vi "F Dwf Analog Out Repeat Info.vi"(7 "pnMax":i32, 8 "error in (no error)":errorcluster, 9 "pnMin":i32, 10 "idxChannel":i32, 11 "hdwf":i32) -> (0 "error out":errorcluster, 1 "pnMin out":i32, 3 "function return":i32, 5 "pnMax out":i32)   [LabVIEW 2021, in "Olasdwf.lvlib"]
doc: "DWFAPI int FDwfAnalogOutRepeatInfo(HDWF hdwf, int idxChannel, int *pnMin, int *pnMax);"
uses:
  Olasdwf.lvlib
  Windows/System32/dwf.dll
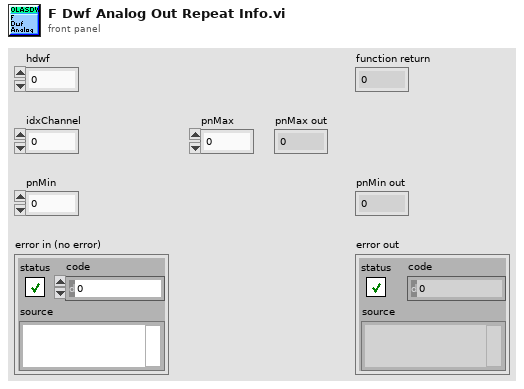
[diagram p1: front panel]
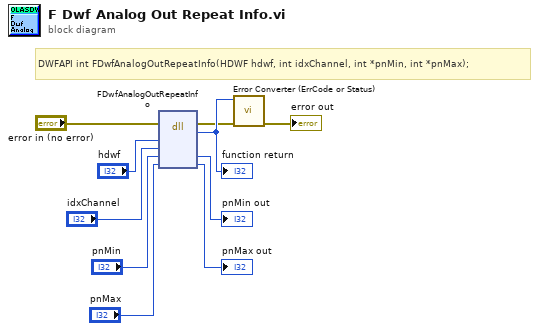
[diagram p0: block diagram]
diagram:
  # "DWFAPI int FDwfAnalogOutRepeatInfo(HDWF hdwf, int idxChannel, int *pnMin, int *pnMax);"
  n1 = dll-call lib="/Windows/System32/dwf.*" fn="FDwfAnalogOutRepeatInfo"(error in="error in (no error)", "hdwf"="hdwf", "idxChannel"="idxChannel", "pnMin"="pnMin", "pnMax"="pnMax") -> (error out=w2:errorcluster, w10:i32, "pnMin"=→"pnMin out":i32, "pnMax"=→"pnMax out":i32)  [unwired: 4 in, 1 out]
  "function return" <- w10
  n2 = call "Error Converter (ErrCode or Status).vi"("error in (no error)"=w2, "error code"=w10) -> ("error out"=→"error out":errorcluster)  [unwired: 9 in]
